vi "Seven Segment Write Char.vi"(0 "Arduino Resource":T1={"VISA resource"="", "Board Type"=enum."Uno", "Connection Type"=enum."USB / Serial", "Bytes Per Packet (15)"=15}, 7 "Character":string, 11 "error in (no error)":errorcluster) -> (4 "Arduino Resource":T1={"VISA resource"="", "Board Type"=enum."Uno", "Connection Type"=enum."USB / Serial", "Bytes Per Packet (15)"=15}, 15 "error out":errorcluster)   [LabVIEW 2015, in "LabVIEW Interface for Arduino.lvlib"]
doc: "Write a single charater to the seven segment display. Arduino Seven Segment Configure must be called to configure the seven segment display pins before calling this VI."
uses:
  <vilib>/LabVIEW Interface for Arduino/LabVIEW Interface for Arduino.lvlib
  <vilib>/LabVIEW Interface for Arduino/Type Defs/Arduino Resource.ctl
  <vilib>/LabVIEW Interface for Arduino/Type Defs/Board Type.ctl
  <vilib>/LabVIEW Interface for Arduino/Type Defs/Command.ctl
  <vilib>/LabVIEW Interface for Arduino/Type Defs/Value.ctl
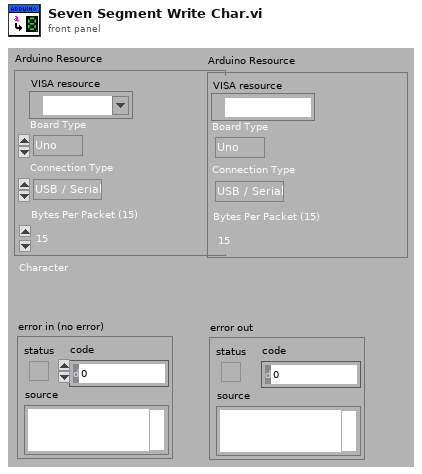
[diagram p1: front panel]
types:
  T1 = typedef "LabVIEW Interface for Arduino.lvlib/Arduino Resource.ctl" = cluster{"VISA resource":refnum<visa-resource-name>, "Board Type":T2, "Connection Type":enum8{"USB / Serial"}, "Bytes Per Packet (15)":u8}
  T2 = typedef "LabVIEW Interface for Arduino.lvlib/Board Type.ctl" = enum16{"Uno", "Dimuelanove w/Atmega 328", "Mega 2560"}
  T3 = typedef "LabVIEW Interface for Arduino.lvlib/Command.ctl" = enum8{"setArduinoMode", "flushSerial", "setPinMode", "digitalWritePin", "digitalWritePort", "tone", "digitalReadPin", "digitalReadPort", "analogReadPin", "analogReadPort", "pwmWritePin", "pwmWritePort", "sevenSegment_Configure", "sevenSegment_Write", "I2C Init", "I2C Write", "I2C Read", "SPI Init", "SPI Set Bit Order", "SPI Set Clock Divider", "SPI Set Data Mode", "SPI Send / Receive", "SPI Close", "Servo Set Num Servos", "Servo Config Servo", "Servo Write Angle", "Servo Read Angle", "Servo Write Pulse Width", "Servo Read Pulse Width", "Servo Detach", "LCD Init", "LCD Set Size", "LCD Set Cursor Mode", "LCD Clear", "LCD Set Cursor Position", "LCD Print", "LCD Display Power", "LCD Scroll Display", "LCD Autoscroll", "LCD Print Direction", "LCD Create Custom Char", "LCD Print Custom Char", "contAcqOn", "contAcqOff", "getFirmwareVersion", "FiniteSampleStart"}
  T4 = typedef "LabVIEW Interface for Arduino.lvlib/Value.ctl" = enum8{"Low", "High"}
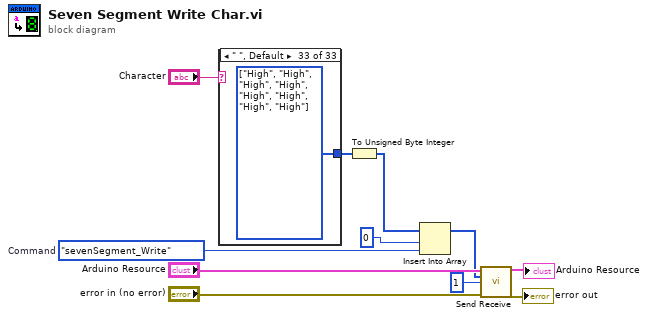
[diagram p0: block diagram]
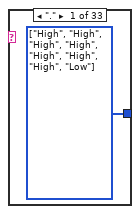
[diagram p2: hidden frame]
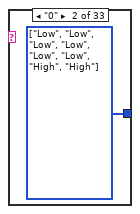
[diagram p3: hidden frame]
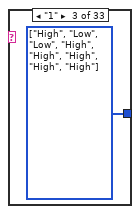
[diagram p4: hidden frame]
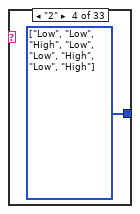
[diagram p5: hidden frame]
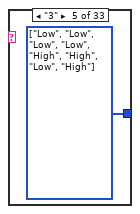
[diagram p6: hidden frame]
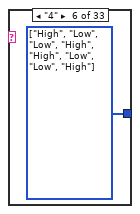
[diagram p7: hidden frame]
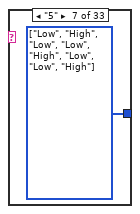
[diagram p8: hidden frame]
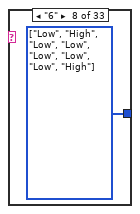
[diagram p9: hidden frame]
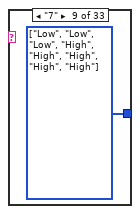
[diagram p10: hidden frame]
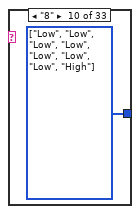
[diagram p11: hidden frame]
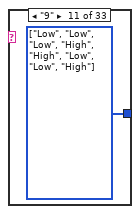
[diagram p12: hidden frame]
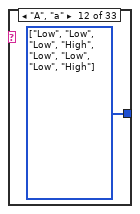
[diagram p13: hidden frame]
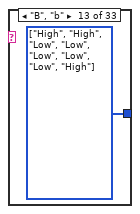
[diagram p14: hidden frame]
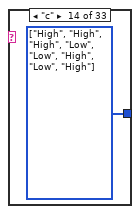
[diagram p15: hidden frame]
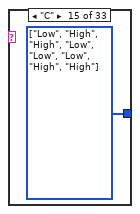
[diagram p16: hidden frame]
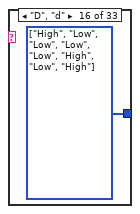
[diagram p17: hidden frame]
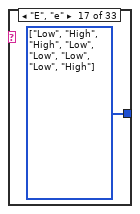
[diagram p18: hidden frame]
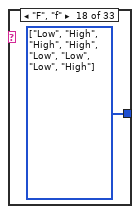
[diagram p19: hidden frame]
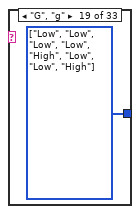
[diagram p20: hidden frame]
diagram:
  w7 = Command."sevenSegment_Write"  # Command
  n1 = case shown="\" \", Default" "Character" {
    tunnel: [w12 w13 w14 w15 w16 w17 w18 w19 w20 w21 w22 w23 w24 w25 w26 w27 w28 w29 w30 w31 w32 w33 w34 w35 w36 w37 w38 w39 w40 w41 w42 w43 w44] -> w9
    frame "." {
      w12 = T4[] [enum."High", enum."High", enum."High", enum."High", enum."High", enum."High", enum."High", enum."Low"] items=["Low", "High"] ("Seven Segment Pins 2")
    }
    frame "0" {
      w13 = T4[] [enum."Low", enum."Low", enum."Low", enum."Low", enum."Low", enum."Low", enum."High", enum."High"] items=["Low", "High"] ("Seven Segment Pins 2")
    }
    frame "1" {
      w14 = T4[] [enum."High", enum."Low", enum."Low", enum."High", enum."High", enum."High", enum."High", enum."High"] items=["Low", "High"] ("Seven Segment Pins 2")
    }
    frame "2" {
      w15 = T4[] [enum."Low", enum."Low", enum."High", enum."Low", enum."Low", enum."High", enum."Low", enum."High"] items=["Low", "High"] ("Seven Segment Pins 2")
    }
    frame "3" {
      w16 = T4[] [enum."Low", enum."Low", enum."Low", enum."Low", enum."High", enum."High", enum."Low", enum."High"] items=["Low", "High"] ("Seven Segment Pins 2")
    }
    frame "4" {
      w17 = T4[] [enum."High", enum."Low", enum."Low", enum."High", enum."High", enum."Low", enum."Low", enum."High"] items=["Low", "High"] ("Seven Segment Pins 2")
    }
    frame "5" {
      w18 = T4[] [enum."Low", enum."High", enum."Low", enum."Low", enum."High", enum."Low", enum."Low", enum."High"] items=["Low", "High"] ("Seven Segment Pins 2")
    }
    frame "6" {
      w19 = T4[] [enum."Low", enum."High", enum."Low", enum."Low", enum."Low", enum."Low", enum."Low", enum."High"] items=["Low", "High"] ("Seven Segment Pins 2")
    }
    frame "7" {
      w20 = T4[] [enum."Low", enum."Low", enum."Low", enum."High", enum."High", enum."High", enum."High", enum."High"] items=["Low", "High"] ("Seven Segment Pins 2")
    }
    frame "8" {
      w21 = T4[] [enum."Low", enum."Low", enum."Low", enum."Low", enum."Low", enum."Low", enum."Low", enum."High"] items=["Low", "High"] ("Seven Segment Pins 2")
    }
    frame "9" {
      w22 = T4[] [enum."Low", enum."Low", enum."Low", enum."High", enum."High", enum."Low", enum."Low", enum."High"] items=["Low", "High"] ("Seven Segment Pins 2")
    }
    frame "A", "a" {
      w23 = T4[] [enum."Low", enum."Low", enum."Low", enum."High", enum."Low", enum."Low", enum."Low", enum."High"] items=["Low", "High"] ("Seven Segment Pins 2")
    }
    frame "B", "b" {
      w24 = T4[] [enum."High", enum."High", enum."Low", enum."Low", enum."Low", enum."Low", enum."Low", enum."High"] items=["Low", "High"] ("Seven Segment Pins 2")
    }
    frame "c" {
      w25 = T4[] [enum."High", enum."High", enum."High", enum."Low", enum."Low", enum."High", enum."Low", enum."High"] items=["Low", "High"] ("Seven Segment Pins 2")
    }
    frame "C" {
      w26 = T4[] [enum."Low", enum."High", enum."High", enum."Low", enum."Low", enum."Low", enum."High", enum."High"] items=["Low", "High"] ("Seven Segment Pins 2")
    }
    frame "D", "d" {
      w27 = T4[] [enum."High", enum."Low", enum."Low", enum."Low", enum."Low", enum."High", enum."Low", enum."High"] items=["Low", "High"] ("Seven Segment Pins 2")
    }
    frame "E", "e" {
      w28 = T4[] [enum."Low", enum."High", enum."High", enum."Low", enum."Low", enum."Low", enum."Low", enum."High"] items=["Low", "High"] ("Seven Segment Pins 2")
    }
    frame "F", "f" {
      w29 = T4[] [enum."Low", enum."High", enum."High", enum."High", enum."Low", enum."Low", enum."Low", enum."High"] items=["Low", "High"] ("Seven Segment Pins 2")
    }
    frame "G", "g" {
      w30 = T4[] [enum."Low", enum."Low", enum."Low", enum."Low", enum."High", enum."Low", enum."Low", enum."High"] items=["Low", "High"] ("Seven Segment Pins 2")
    }
    frame "h" {
      w31 = T4[] [enum."High", enum."High", enum."Low", enum."High", enum."Low", enum."Low", enum."Low", enum."High"] items=["Low", "High"] ("Seven Segment Pins 2")
    }
    frame "H" {
      w32 = T4[] [enum."High", enum."Low", enum."Low", enum."High", enum."Low", enum."Low", enum."Low", enum."High"] items=["Low", "High"] ("Seven Segment Pins 2")
    }
    frame "I", "i" {
      w33 = T4[] [enum."High", enum."Low", enum."Low", enum."High", enum."High", enum."High", enum."High", enum."High"] items=["Low", "High"] ("Seven Segment Pins 2")
    }
    frame "J", "j" {
      w34 = T4[] [enum."High", enum."Low", enum."Low", enum."Low", enum."Low", enum."High", enum."High", enum."High"] items=["Low", "High"] ("Seven Segment Pins 2")
    }
    frame "L", "l" {
      w35 = T4[] [enum."High", enum."High", enum."High", enum."Low", enum."Low", enum."Low", enum."High", enum."High"] items=["Low", "High"] ("Seven Segment Pins 2")
    }
    frame "N", "n" {
      w36 = T4[] [enum."High", enum."High", enum."Low", enum."High", enum."Low", enum."High", enum."Low", enum."High"] items=["Low", "High"] ("Seven Segment Pins 2")
    }
    frame "O" {
      w37 = T4[] [enum."Low", enum."Low", enum."Low", enum."Low", enum."Low", enum."Low", enum."High", enum."High"] items=["Low", "High"] ("Seven Segment Pins 2")
    }
    frame "o" {
      w38 = T4[] [enum."High", enum."High", enum."Low", enum."Low", enum."Low", enum."High", enum."Low", enum."High"] items=["Low", "High"] ("Seven Segment Pins 2")
    }
    frame "P", "p" {
      w39 = T4[] [enum."Low", enum."Low", enum."High", enum."High", enum."Low", enum."Low", enum."Low", enum."High"] items=["Low", "High"] ("Seven Segment Pins 2")
    }
    frame "S", "s" {
      w40 = T4[] [enum."Low", enum."High", enum."Low", enum."Low", enum."High", enum."Low", enum."Low", enum."High"] items=["Low", "High"] ("Seven Segment Pins 2")
    }
    frame "u" {
      w41 = T4[] [enum."High", enum."High", enum."Low", enum."Low", enum."Low", enum."High", enum."High", enum."High"] items=["Low", "High"] ("Seven Segment Pins 2")
    }
    frame "U" {
      w42 = T4[] [enum."High", enum."Low", enum."Low", enum."Low", enum."Low", enum."Low", enum."High", enum."High"] items=["Low", "High"] ("Seven Segment Pins 2")
    }
    frame "Y", "y" {
      w43 = T4[] [enum."High", enum."Low", enum."Low", enum."Low", enum."High", enum."Low", enum."Low", enum."High"] items=["Low", "High"] ("Seven Segment Pins 2")
    }
    frame " ", Default {
      w44 = T4[] [enum."High", enum."High", enum."High", enum."High", enum."High", enum."High", enum."High", enum."High"] items=["Low", "High"] ("Seven Segment Pins 2")
    }
  }
  n2 = To Unsigned Byte Integer(number=w9) -> (unsigned 8bit integer=w8:u8[])
  n3 = Insert Into Array(array=w8, index=0, new element=w7) -> (w2:u8[])
  n4 = call <vilib>:"Send Receive.vi"("Arduino Resource"="Arduino Resource", "Data"=w2, "Bytes To Read (0)"=u32 1, "error in"="error in (no error)") -> ("Arduino Resource"=→"Arduino Resource":T1, "error out"=→"error out":errorcluster)  [unwired: 9 in, 1 out]
